vi "Start livestream video from CamServer (TCP CLIENT).vi"(0 "TCP/IP port":u16=80, 1 "Camera":T2="Travcam", 2 "Write video":bool, 3 "Video directory path":path, 4 "Video name":string) -> (5 "Error out":errorcluster)   [LabVIEW 2015]
doc: "Starts a video livestream from the camera server. The stream can also be saved to a local directory."
uses:
  Camera enum/Camera enum.ctl
  <vilib>/vision/Avi.llb/IMAQ AVI2 Refnum.ctl
  Globals/CamServer global.vi
panel:
  in  "Stop":bool
  out "Video":T1(plugin-control)
  # "PN 25/08/15"
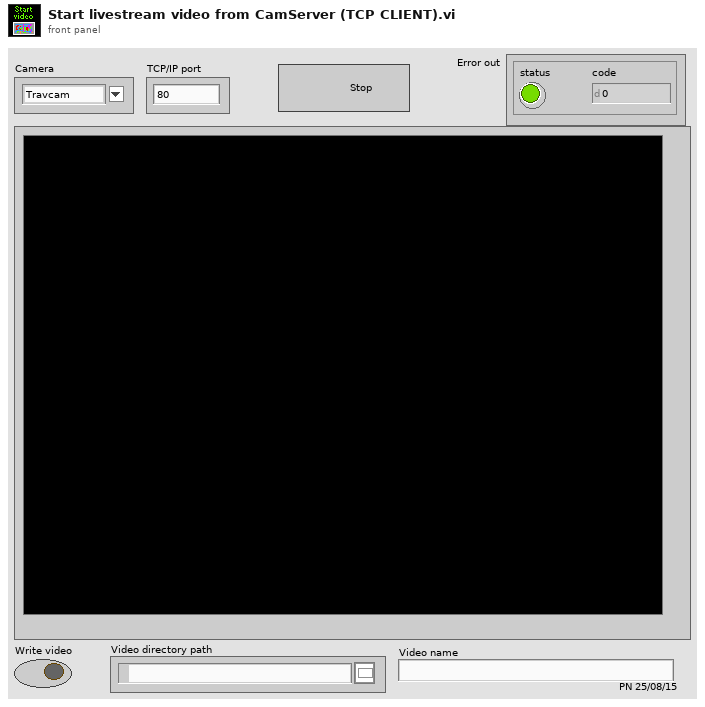
[diagram p1: front panel]
types:
  T1 = typedef "IMAQ Image.ctl" = refnum<image>
  T2 = typedef "Camera enum.ctl" = string
  T3 = typedef "IMAQ AVI2 Refnum.ctl" = refnum<k20>
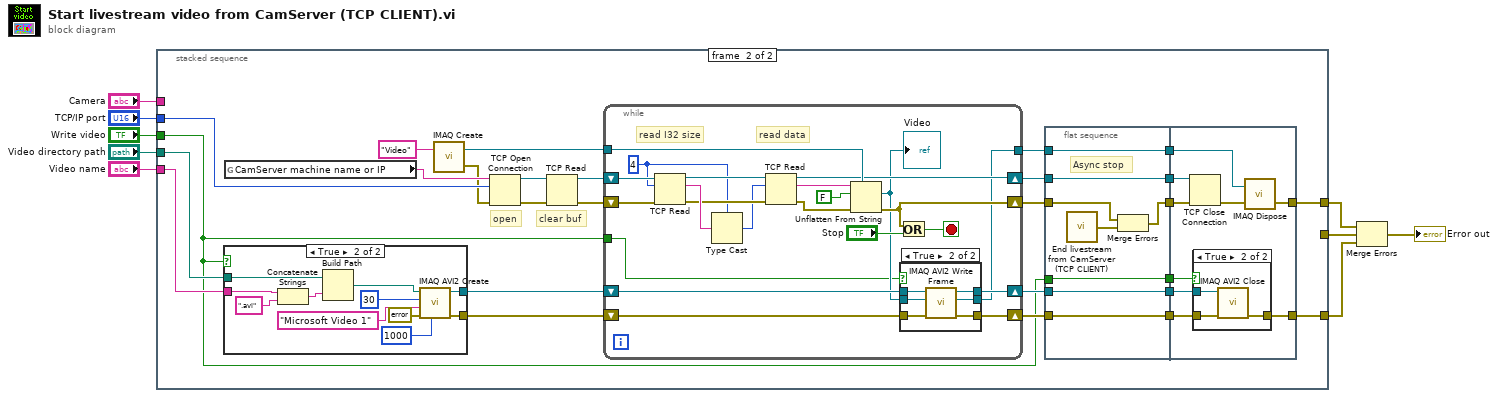
[diagram p0: block diagram]
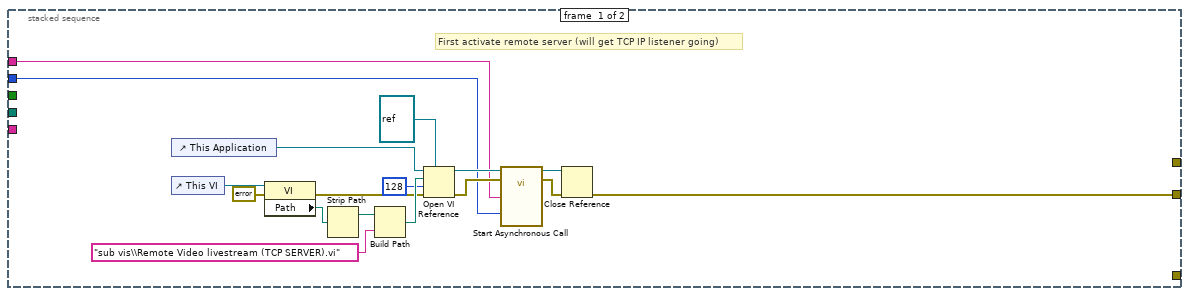
[diagram p2: hidden frame]
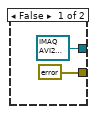
[diagram p3: hidden frame]
diagram:
  n1 = stacked-sequence {
    tunnel: "Camera" -> [w12 _]
    tunnel: "TCP/IP port" -> [w11 w53]
    tunnel: "Write video" -> [_ w28]
    tunnel: [w10 _] -> w6
    tunnel: [_ w38] -> w5
    tunnel: [_ w31] -> w3
    tunnel: "Video name" -> [_ w30]
    tunnel: "Video directory path" -> [_ w29]
    frame #0 {
      # "First activate remote server (will get TCP IP listener going)"
      n2 = control-ref of="This Application"() -> (w21:refnum<vi>)
      n3 = control-ref of="This VI"() -> (w26:refnum<vi>)
      n4 = property class="VI"(reference=w26, error in=errorcluster {"status"=FALSE, "code"=0, "source"=""} ("error in (no error)")) -> (error out=w23:errorcluster, "Path"=w19:path)  [unwired: 1 out]
      n5 = Strip Path(path=w19) -> (stripped path=w18:path)  [unwired: 1 out]
      n6 = Build Path(base path=w18, name or relative path="sub vis\\Remote Video livestream (TCP SERVER).vi") -> (appended path=w24:path)
      n7 = Open VI Reference(type specifier VI Refnum (for type only)=refnum<vi> refnum, application reference (local)=w21, vi path=w24, options=128, error in (no error)=w23) -> (vi reference=w17:refnum<vi>, error out=w16:errorcluster)  [unwired: 1 in]
      n8 = call-by-ref "Start Asynchronous Call"(reference=w17, error in=w16, "TCP/IP port"=w11, "Camera"=w12) -> (reference out=w14:refnum<vi>, error out=w13:errorcluster)  [unwired: 1 out]
      n9 = Close Reference(reference=w14, error in (no error)=w13) -> (error out=w10:errorcluster)
    }
    frame #1 {
      # "open"
      # "clear buf"
      n10 = case shown="True" w28 {
        tunnel: [T3 refnum ("AVI Refnum") w65] -> w37
        tunnel: [errorcluster {"status"=FALSE, "code"=0, "source"=""} ("error out") w64] -> w36
        tunnel: w30 -> [_ w57]
        tunnel: w29 -> [_ w56]
        frame False {
        }
        frame True {
          n11 = Concatenate Strings(w57, ".avi" ("name or relative path")) -> (w59:string)
          n12 = Build Path(base path=w56, name or relative path=w59) -> (appended path=w58:path)
          n13 = call "IMAQ AVI2 Create"("Quality"=1000, "error in (no error)"=errorcluster {"status"=FALSE, "code"=0, "source"=""} ("error in"), "Codec"="Microsoft Video 1", "Frames Per Second"=u32 30, "AVI Path"=w58) -> ("error out"=w64:errorcluster, "AVI Refnum"=w65:T3)  [unwired: 5 in]
        }
      }
      n14 = global read "CamServer global.vi" "CamServer machine name or IP"() -> (w52:string)
      n15 = call "IMAQ Create"("Image Name"="Video") -> ("New Image"=w46:T1, "error out"=w45:errorcluster)  [unwired: 4 in]
      n16 = TCP Open Connection(address=w52, remote port or service name=w53, error in (no error)=w45) -> (connection ID=w50:refnum<k5>, error out=w51:errorcluster)  [unwired: 2 in]
      n17 = TCP Read(connection ID=w50, error in (no error)=w51) -> (connection ID out=w48:refnum<k5>, error out=w49:errorcluster)  [unwired: 3 in, 1 out]
      n18 = while {
        shift-right: [w98] -> w44
        shift-left: w48 -> [w109]
        shift-right: [w97] -> w43
        shift-left: w49 -> [w107]
        tunnel: w46 -> [w100]
        tunnel: [w88] -> w42
        shift-right: [w92] -> w32
        shift-left: w36 -> [w91]
        shift-right: [w93] -> w35
        shift-left: w37 -> [w94]
        tunnel: w28 -> [w89]
        stop <- w95 stop-if-true
        w99 = 4
        # "read data"
        # "read I32 size"
        n19 = TCP Read(connection ID=w109, bytes to read=w99, error in (no error)=w107) -> (connection ID out=w106:refnum<k5>, data out=w108:string, error out=w105:errorcluster)  [unwired: 2 in]
        n20 = Type Cast(type=w99, x=w108) -> (*(type *) &x=w104:i32)
        n21 = TCP Read(connection ID=w106, bytes to read=w104, error in (no error)=w105) -> (connection ID out=w98:refnum<k5>, data out=w103:string, error out=w101:errorcluster)  [unwired: 2 in]
        n22 = Unflatten From String(type=w100, binary string=w103, data includes array or string size? (T)=FALSE, error in (no error)=w101) -> (value=w90:T1, error out=w97:errorcluster)  [unwired: 1 in, 1 out]
        "Video" <- w90
        n23 = Or(x=w97, y="Stop") -> (x .or. y?=w95:bool)
        n24 = case shown="True" w89 {
          tunnel: w94 -> [w112 w118]
          tunnel: w90 -> [w110 w117]
          tunnel: [w112 w116] -> w93
          tunnel: [w111 w115] -> w92
          tunnel: w91 -> [w111 w114]
          tunnel: [w110 w113] -> w88
          frame False {
          }
          frame True {
            n25 = call "IMAQ AVI2 Write Frame"("error in (no error)"=w114, "Image"=w117, "AVI Refnum"=w118) -> ("error out"=w115:errorcluster, "Image Out (duplicate)"=w113:T1, "AVI Refnum (duplicate)"=w116:T3)  [unwired: 6 in]
          }
        }
      }
      n26 = flat-sequence {
        tunnel: w42 -> [w73]
        tunnel: w43 -> [w71]
        tunnel: w44 -> [w74]
        tunnel: [w74] -> w41
        tunnel: [w70] -> w40
        tunnel: [w73] -> w39
        tunnel: w35 -> [w69]
        tunnel: [w69] -> w34
        tunnel: w32 -> [w68]
        tunnel: [w68] -> w33
        tunnel: w28 -> [w67]
        tunnel: [w67] -> w27
        tunnel: w41 -> [w83]
        tunnel: w40 -> [w82]
        tunnel: w39 -> [w80]
        tunnel: [w79] -> w38
        tunnel: w34 -> [w78]
        tunnel: w33 -> [w77]
        tunnel: [w76] -> w31
        tunnel: w27 -> [w75]
        frame #0 {
          # "Async stop"
          n27 = call "End livestream from CamServer (TCP CLIENT).vi"() -> ("Error out"=w72:errorcluster)  [unwired: 1 in]
          n28 = Merge Errors(w71, w72) -> (w70:errorcluster)
        }
        frame #1 {
          n29 = TCP Close Connection(connection ID=w83, error in (no error)=w82) -> (error out=w81:errorcluster)  [unwired: 1 in, 1 out]
          n30 = case shown="True" w75 {
            tunnel: w77 -> [w84 w87]
            tunnel: [w84 w86] -> w76
            tunnel: w78 -> [_ w85]
            frame False {
            }
            frame True {
              n31 = call "IMAQ AVI2 Close"("error in (no error)"=w87, "AVI Refnum"=w85) -> ("error out"=w86:errorcluster)  [unwired: 9 in]
            }
          }
          n32 = call "IMAQ Dispose"("Image"=w80, "error in (no error)"=w81) -> ("error out"=w79:errorcluster)  [unwired: 4 in]
        }
      }
    }
  }
  n33 = Merge Errors(w5, w6, w3) -> (→"Error out":errorcluster)
